vi "SetDateOfBirth.vi"(8 "Error In":errorcluster, 10 "DateOfBirth":timestamp, 11 "reference in":refnum<class "Customer.lvclass">) -> (0 "Error Out":errorcluster, 3 "reference out":refnum<class "Customer.lvclass">)   [LabVIEW 2020, in "Customer.lvclass"]
uses:
  Customer.lvclass
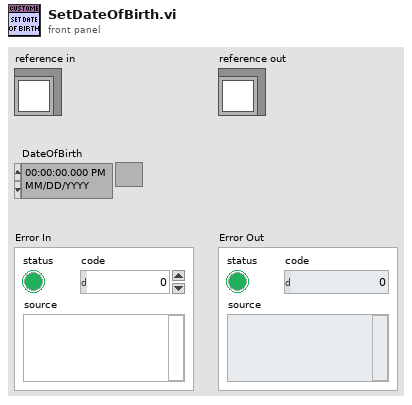
[diagram p1: front panel]
types:
  T1 = typedef "Customer.lvclass/ObjectAttributes.ctl" = cluster{"DateOfFirstPurchase":timestamp, "DateOfBirth":timestamp, "IsVeteran":bool, "Referrer":refnum<class "ReferredBy.lvclass">}
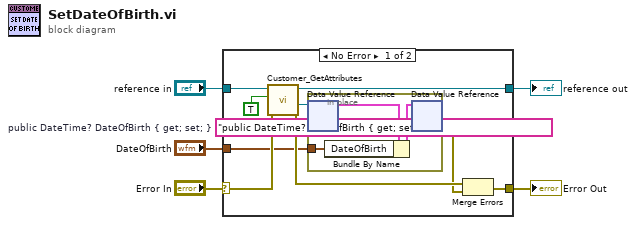
[diagram p0: block diagram]
diagram:
  (unwired) "public DateTime? DateOfBirth { get; set; }"  # public DateTime? DateOfBirth { get; set; }
  n1 = case shown="No Error" "Error In" {
    selector: "Error In" -> [w13 w19]
    tunnel: [w14 w19] -> w4
    tunnel: [w10 w18] -> w2
    tunnel: "reference in" -> [w11 w18]
    tunnel: "DateOfBirth" -> [w7 _]
    frame No Error {
      n2 = call "Customer_GetAttributes.vi"("error in (no error)"=w13, "OnlyGetDvrReference(False)"=TRUE, "reference in"=w11) -> ("error out"=w12:errorcluster, "DataRef"=w8:refnum<data-value>, "reference out"=w10:refnum<class "Customer.lvclass">)  [unwired: 5 in, 1 out]
      n3 = in-place {
        in-place-border: w7 -> [w17]
        n4 = in-place-dvr #1(w8) -> (w16:T1)  [unwired: 1 out]
        n5 = Bundle By Name(cluster=w16, "DateOfBirth"=w17) -> (w15:T1)
        n6 = in-place-dvr #1(w15) -> (w6:errorcluster)  [unwired: 1 out]
      }
      n7 = Merge Errors(w12, w6) -> (w14:errorcluster)
    }
    frame Error {
    }
  }
  "Error Out" <- w4
  "reference out" <- w2
